vi "Quantum Composers 9000 Series Recall-Save Configuration.vi"() -> ()   [LabVIEW 2012]
doc: "This VI is an example of how to use subVIs from the QC 9000 series driver to programmatically recall/save a configuration from/to the unit's non-volatile memory.\n\n\nNotes:\n1) The pulse generator keypad is returned to \"Local\" mode when this VI terminates in order to restore manual control to the user.\n2) VISA Version 3.3 or higher must be installed to use this instrument driver."
uses:
  Support/Channel Parameters.ctl
  Support/System Parameters.ctl
  Quantum Composers 9000 Series.lvlib
panel:
  in  "Write data \n(off reads data)":bool=TRUE
  in  "Memory  (1)":i32=1
  in  "System Parameters":T1={"Sys Period"=0.000142, "Sys Mode"=enum."Normal", "Sys Burst #"=4, "Sys DC On"=3, "Sys DC Off"=2, "Sys State"=TRUE, "Sys Gate"=FALSE, "Sys Trig Edge"=TRUE, "Sys Ext Mode"=enum."Disabled", "Sys Trig Lev"=2.5, "Sys Gate Lev "=0.0, "Sys Gate Mode"=enum."Disabled"} {"Sys Gate Lev" format="%.4p"; "Sys Trig Lev" format="%.4p"; "Sys Period" format="%.6p"}
  in  "VISA resource":refnum<visa-resource-name>="QCpulseGen"
  in  "Channel Parameters":T2[](array[typedef])=[{"Channel"=1, "Chan State"=TRUE, "Chan Sync Source"=0, "Chan Gate Logic"=enum."Disabled", "Chan Mode"=enum."Normal", "Chan Wait #"=0, "Chan Delay"=2e-07, "Chan Width"=1e-06, "Chan Burst #"=5, "Chan DC On"=4, "Chan DC Off"=3, "Chan Polarity"=FALSE, "Chan MUX Value"=1, "Chan Level Out"=enum."TTL", "Chan Lev Adjust"=9.0, "Chan Gate Mode"=enum."Disabled"}, {"Channel"=2, "Chan State"=TRUE, "Chan Sync Source"=0, "Chan Gate Logic"=enum."Disabled", "Chan Mode"=enum."Normal", "Chan Wait #"=0, "Chan Delay"=1.25e-06, "Chan Width"=1e-06, "Chan Burst #"=5, "Chan DC On"=4, "Chan DC Off"=3, "Chan Polarity"=FALSE, "Chan MUX Value"=2, "Chan Level Out"=enum."TTL", "Chan Lev Adjust"=5.0, "Chan Gate Mode"=enum."Disabled"}, {"Channel"=3, "Chan State"=TRUE, "Chan Sync Source"=0, "Chan Gate Logic"=enum."Disabled", "Chan Mode"=enum."Duty Cycle", "Chan Wait #"=0, "Chan Delay"=2e-07, "Chan Width"=0.00994, "Chan Burst #"=5, "Chan DC On"=1, "Chan DC Off"=139, "Chan Polarity"=FALSE, "Chan MUX Value"=4, "Chan Level Out"=enum."TTL", "Chan Lev Adjust"=5.0, "Chan Gate Mode"=enum."Disabled"}, {"Channel"=4, "Chan State"=TRUE, "Chan Sync Source"=0, "Chan Gate Logic"=enum."Disabled", "Chan Mode"=enum."Duty Cycle", "Chan Wait #"=0, "Chan Delay"=2e-07, "Chan Width"=0.00994, "Chan Burst #"=5, "Chan DC On"=1, "Chan DC Off"=139, "Chan Polarity"=FALSE, "Chan MUX Value"=8, "Chan Level Out"=enum."TTL", "Chan Lev Adjust"=5.0, "Chan Gate Mode"=enum."Disabled"}, {"Channel"=5, "Chan State"=TRUE, "Chan Sync Source"=0, "Chan Gate Logic"=enum."Disabled", "Chan Mode"=enum."Duty Cycle", "Chan Wait #"=70, "Chan Delay"=2e-07, "Chan Width"=0.00994, "Chan Burst #"=5, "Chan DC On"=1, "Chan DC Off"=139, "Chan Polarity"=FALSE, "Chan MUX Value"=16, "Chan Level Out"=enum."TTL", "Chan Lev Adjust"=5.0, "Chan Gate Mode"=enum."Disabled"}, {"Channel"=6, "Chan State"=TRUE, "Chan Sync Source"=0, "Chan Gate Logic"=enum."Disabled", "Chan Mode"=enum."Duty Cycle", "Chan Wait #"=0, "Chan Delay"=0.0, "Chan Width"=1.2e-06, "Chan Burst #"=5, "Chan DC On"=70, "Chan DC Off"=70, "Chan Polarity"=TRUE, "Chan MUX Value"=32, "Chan Level Out"=enum."TTL", "Chan Lev Adjust"=5.0, "Chan Gate Mode"=enum."Disabled"}, {"Channel"=7, "Chan State"=TRUE, "Chan Sync Source"=0, "Chan Gate Logic"=enum."Disabled", "Chan Mode"=enum."Duty Cycle", "Chan Wait #"=70, "Chan Delay"=0.0, "Chan Width"=1.2e-06, "Chan Burst #"=5, "Chan DC On"=70, "Chan DC Off"=70, "Chan Polarity"=TRUE, "Chan MUX Value"=64, "Chan Level Out"=enum."TTL", "Chan Lev Adjust"=5.0, "Chan Gate Mode"=enum."Disabled"}, {"Channel"=8, "Chan State"=TRUE, "Chan Sync Source"=0, "Chan Gate Logic"=enum."Disabled", "Chan Mode"=enum."Normal", "Chan Wait #"=0, "Chan Delay"=0.0, "Chan Width"=1.35e-06, "Chan Burst #"=5, "Chan DC On"=4, "Chan DC Off"=3, "Chan Polarity"=TRUE, "Chan MUX Value"=128, "Chan Level Out"=enum."Adjustable", "Chan Lev Adjust"=7.0, "Chan Gate Mode"=enum."Disabled"}] {"Chan Sync Source" items=["System (To)", "Channel A", "Channel B", "Channel C", "Channel D", "Channel E", "Channel F", "Channel G", "Channel H"]; "Chan Width" format="%.3p"; "Chan Delay" format="%.3p"; "Chan Lev Adjust" format="%.3p"; "Channel" items=["Channel A"=1, "Channel B"=2, "Channel C"=3, "Channel D"=4, "Channel E"=5, "Channel F"=6, "Channel G"=7, "Channel H"=8]}
  # "9000 Series\nPulse Generator\nExample Program"
  # "Notes:\n1.  The channel parameters \"Burst #\", \"DC On\", \"DC Off\", and \"Adjustable\" are only updated when operating in the corresponding mode.\n2.  The system parameters  \"Burst #\", \"DC On\", \"DC Off\", and \"Trig Level\"` are only updated when operating in the corresponding mode."
  # "Input"
  # "Triggered"
  # "Gated"
  # "Mode"
  # "Burst"
  # "Duty\nCycle"
  # "Input"
  # "Normal\nSingle\nBurst"
  # "Burst"
  # "Duty Cycle"
  # "Output"
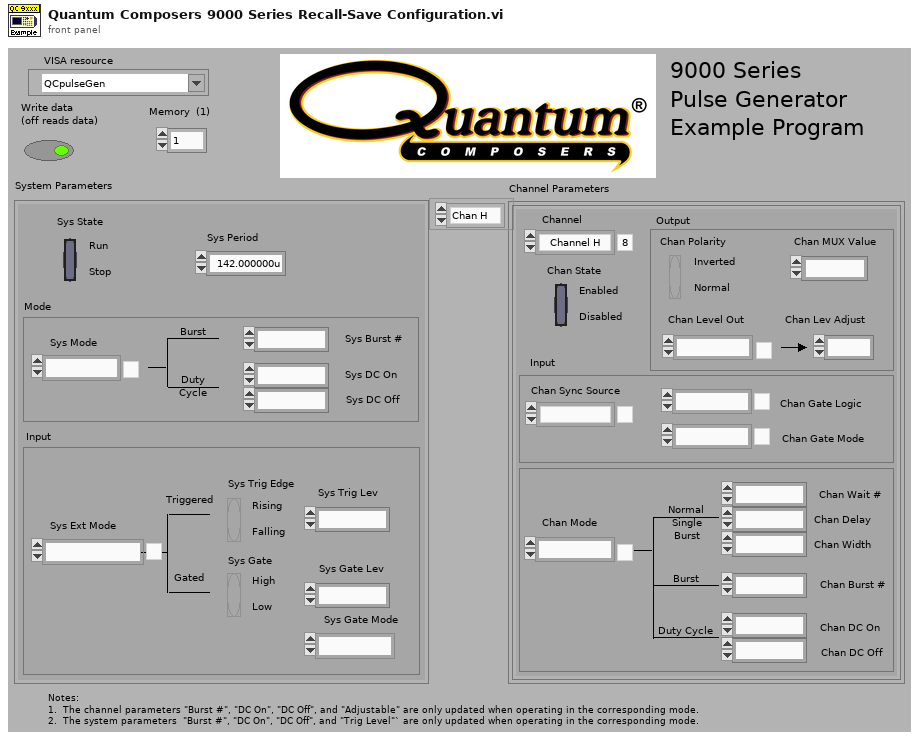
[diagram p1: front panel]
types:
  T1 = typedef "System Parameters.ctl" = cluster{"Sys Period":dbl, "Sys Mode":enum16{"Normal", "Single", "Burst", "Duty Cycle"}, "Sys Burst #":i32, "Sys DC On":i32, "Sys DC Off":i32, "Sys State":bool, "Sys Gate":bool, "Sys Trig Edge":bool, "Sys Ext Mode":enum16{"Disabled", "Triggered", "Gated", "Triggered & Gated"}, "Sys Trig Lev":dbl, "Sys Gate Lev ":dbl, "Sys Gate Mode":enum16{"Disabled", "Pulse Inhibit", "Output Inhibit", "Channel"}}
  T2 = typedef "Channel Parameters.ctl" = cluster{"Channel":i32, "Chan State":bool, "Chan Sync Source":i32, "Chan Gate Logic":enum16{"Disabled", "Low", "High"}, "Chan Mode":enum16{"Normal", "Single", "Burst", "Duty Cycle"}, "Chan Wait #":i32, "Chan Delay":dbl, "Chan Width":dbl, "Chan Burst #":i32, "Chan DC On":i32, "Chan DC Off":i32, "Chan Polarity":bool, "Chan MUX Value":i32, "Chan Level Out":enum16{"TTL", "Adjustable", "35 Volt", "Optical"}, "Chan Lev Adjust":dbl, "Chan Gate Mode":enum16{"Disabled", "Pulse Inhibit", "Output Inhibit"}}
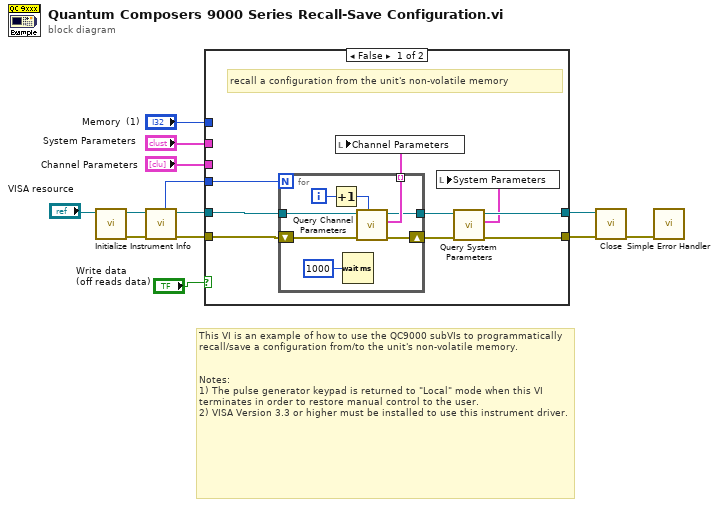
[diagram p0: block diagram]
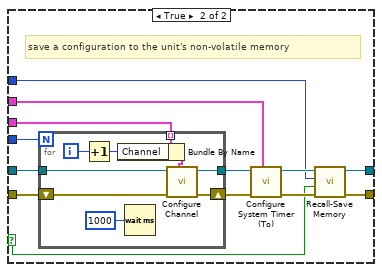
[diagram p2: hidden frame]
diagram:
  # "This VI is an example of how to use the QC9000 subVIs to programmatically recall/save a configuration from/to the unit's non-volatile memory.\n\n\nNotes:\n1) The pulse generator keypad is returned to \"Local\" mode when this VI terminates in order to restore manual control to the user.\n2) VISA Version 3.3 or higher must be installed to use this instrument driver."
  n1 = call "Initialize.vi"("VISA resource name"="VISA resource") -> ("error out"=w7:errorcluster, "VISA resource name out"=w6:refnum<visa-resource-name>)  [unwired: 4 in, 5 out]
  n2 = call "Instrument Info.vi"("error in (no error)"=w7, "VISA resource name"=w6) -> ("error out"=w3:errorcluster, "VISA resource name out"=w4:refnum<visa-resource-name>, "Channels"=w5:i32)  [unwired: 7 out]
  n3 = case shown="False" "Write data \n(off reads data)" {
    selector: "Write data \n(off reads data)" -> [_ w31]
    tunnel: "Channel Parameters" -> [_ w43]
    tunnel: w4 -> [w15 w42]
    tunnel: w3 -> [w14 w41]
    tunnel: "System Parameters" -> [_ w40]
    tunnel: [w19 w35] -> w10
    tunnel: [w18 w34] -> w9
    tunnel: "Memory  (1)" -> [_ w33]
    tunnel: w5 -> [w16 w32]
    frame False {
      # "recall a configuration from the unit's non-volatile memory"
      n4 = for {
        N: w16 -> [_]
        tunnel: w15 -> [w30]
        tunnel: [w29] -> w22 mode=indexing
        shift-right: [w27] -> w20
        shift-left: w14 -> [w28]
        tunnel: [w26] -> w21
        i -> [w25]
        n5 = Increment(x=w25) -> (x+1=w24:i32)
        n6 = Wait (ms)(milliseconds to wait=u32 1000) -> ()  [unwired: 1 out]
        n7 = call "Query Channel Parameters.vi"("Channel (1:Chan A)"=w24, "error in (no error)"=w28, "VISA resource name"=w30) -> ("error out"=w27:errorcluster, "Chan Parameters"=w29:T2, "VISA resource name out"=w26:refnum<visa-resource-name>)  [unwired: 6 out]
      }
      n8 = local write "Channel Parameters"(w22) -> ()
      n9 = call "Query System Parameters.vi"("error in (no error)"=w20, "VISA resource name"=w21) -> ("error out"=w18:errorcluster, "System Parameters"=w17:T1, "VISA resource name out"=w19:refnum<visa-resource-name>)  [unwired: 7 out]
      n10 = local write "System Parameters"(w17) -> ()
    }
    frame True {
      # "save a configuration to the unit's non-volatile memory"
      n11 = for {
        N: w32 -> [_]
        tunnel: [w52] -> w39
        tunnel: w43 -> [w47] mode=indexing
        shift-right: [w51] -> w38
        shift-left: w41 -> [w50]
        tunnel: w42 -> [w49]
        i -> [w46]
        n12 = Increment(x=w46) -> (x+1=w45:i32)
        n13 = Bundle By Name(cluster=w47, "Channel"=w45) -> (w48:T2)
        n14 = Wait (ms)(milliseconds to wait=u32 1000) -> ()  [unwired: 1 out]
        n15 = call "Configure Channel.vi"("Chan Parameters"=w48, "error in (no error)"=w50, "VISA resource name"=w49) -> ("error out"=w51:errorcluster, "VISA resource name out"=w52:refnum<visa-resource-name>)  [unwired: 7 out]
      }
      n16 = call "Configure System Timer (To).vi"("System Parameters"=w40, "error in (no error)"=w38, "VISA resource name"=w39) -> ("error out"=w36:errorcluster, "VISA resource name out"=w37:refnum<visa-resource-name>)  [unwired: 7 out]
      n17 = call "Recall-Save Memory.vi"("error in (no error)"=w36, "Recall/Save (F:Read)"=w31, "Memory  (1)"=w33, "VISA resource name"=w37) -> ("error out"=w34:errorcluster, "VISA resource name out"=w35:refnum<visa-resource-name>)  [unwired: 6 out]
    }
  }
  n18 = call "Close.vi"("error in (no error)"=w9, "VISA resource name"=w10) -> ("error out"=w2:errorcluster)  [unwired: 9 out]
  n19 = call <vilib>:"Simple Error Handler.vi"("error in (no error)"=w2) -> ()  [unwired: 1 in, 8 out]
